vi "set or clear phys units.vi"(4 "zero interval (s)":dbl=1.0 min=1.0 format="%.1f", 5 "Data frequency":ext=1.0 format="%.2f", 6 "History Data":sgl[][](array[numeric]) format="%.2f", 7 "calibration":T3(array[cluster]) {"target value" format="%.2f"}) -> (3 "calibration out":T3(array[cluster]) {"target value" format="%.2f"})   [LabVIEW 2012]
uses:
  TCP DAQ/Set.ctl
  TCP DAQ/clear offset.ctl
  <vilib>/Analysis/baseanly.llb/Mean (DBL).vi
  <vilib>/Analysis/NI_AALBase.lvlib
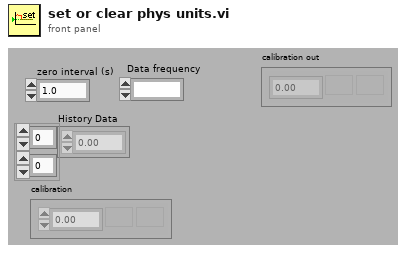
[diagram p1: front panel]
types:
  T1 = typedef "Set.ctl" = bool
  T2 = typedef "clear offset.ctl" = bool
  T3 = cluster{"Set":T1, "target value":dbl, "Clear":T2}[]
  T4 = cluster{"Set":T1, "target value":dbl, "Clear":T2}
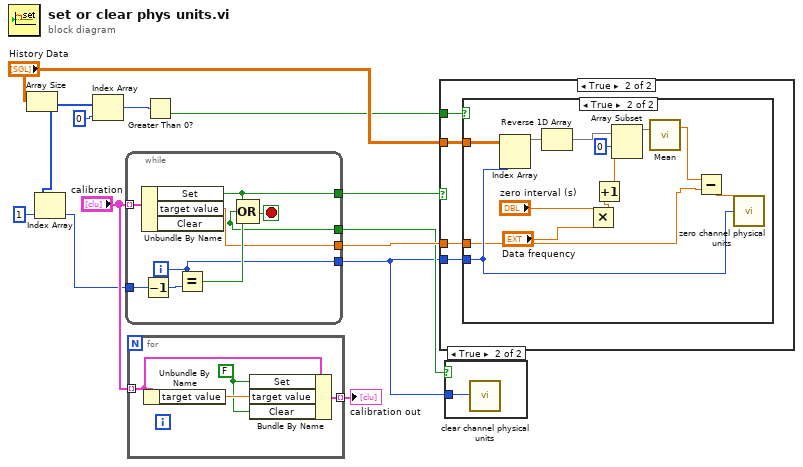
[diagram p0: block diagram]
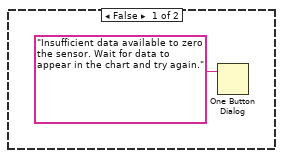
[diagram p4: hidden frame]
diagram:
  n1 = Array Size(array="History Data") -> (size(s)=w12:i32[])
  n2 = Index Array(array=w12, index=1) -> (element=w4:i32)
  n3 = Index Array(array=w12, index=0) -> (element=w3:i32)
  n4 = while {
    tunnel: "calibration" -> [w16] mode=indexing
    tunnel: w4 -> [w21]
    tunnel: [w18] -> w1
    tunnel: [w17] -> w9
    tunnel: [w15] -> w10
    tunnel: [w14] -> w2
    i -> [w18]
    stop <- w22 stop-if-true
    n5 = Unbundle By Name(w16) -> ("Set"=w17:T1, "target value"=w15:dbl, "Clear"=w14:T2)
    n6 = Decrement(x=w21) -> (x-1=w20:i32)
    n7 = Equal?(x=w18, y=w20) -> (x = y?=w19:bool)
    n8 = Compound Arithmetic op=OR(w17, w14, w19) -> (w22:T1)
  }
  n9 = for {
    tunnel: "calibration" -> [w26] mode=indexing
    tunnel: [w23] -> w7 mode=indexing
    w24 = T1 FALSE ("Set")
    n10 = Unbundle By Name(w26) -> ("target value"=w25:dbl)
    n11 = Bundle By Name(cluster=w26, "Set"=w24, "target value"=w25, "Clear"=w24) -> (w23:T4)
  }
  "calibration out" <- w7
  n12 = Greater Than 0?(x=w3) -> (x > 0?=w6:bool)
  n13 = case shown="True" w9 {
    tunnel: "History Data" -> [_ w30]
    tunnel: w1 -> [_ w29]
    tunnel: w10 -> [_ w28]
    tunnel: w6 -> [_ w27]
    frame False {
    }
    frame True {
      n14 = case shown="True" w27 {
        tunnel: w30 -> [_ w37]
        tunnel: w29 -> [_ w34]
        tunnel: w28 -> [_ w32]
        frame False {
          n15 = One Button Dialog(message="Insufficient data available to zero the sensor. Wait for data to appear in the chart and try again.") -> ()  [unwired: 1 in, 1 out]
        }
        frame True {
          n16 = Index Array(array=w37, index (col)=w34) -> (element=w43:sgl[])  [unwired: 1 in]
          n17 = Reverse 1D Array(array=w43) -> (reversed array=w42:sgl[])
          n18 = Multiply(x="zero interval (s)", y="Data frequency") -> (x*y=w39:ext)
          n19 = Increment(x=w39) -> (x+1=w35:ext)
          n20 = Array Subset(array=w42, index=0, length=w35) -> (w44:sgl[])
          n21 = call-poly <vilib>:"Mean.vi"("X"=w44) -> ("mean"=w33:dbl)  [unwired: 1 out]
          n22 = Subtract(x=w33, y=w32) -> (x-y=w36:dbl)
          n23 = call "zero channel physical units.vi"("Index"=w34, "Mean (physical units)"=w36) -> ()  [unwired: 6 in]
        }
      }
    }
  }
  n24 = case shown="True" w2 {
    tunnel: w1 -> [_ w45]
    frame False {
    }
    frame True {
      n25 = call "clear channel physical units.vi"("Index"=w45) -> ()  [unwired: 7 in]
    }
  }
